vi "Image Display Loop.vi"(11 "Notifier in":refnum<notifier>) -> ()   [LabVIEW 2015]
uses:
  <vilib>/vision/Image Controls.llb/IMAQ Image.ctl
  <vilib>/vision/NI_Vision_Development_Module.lvlib
panel:
  out "Display":T1(plugin-control)
  out "Waveform Graph":T2(graph)
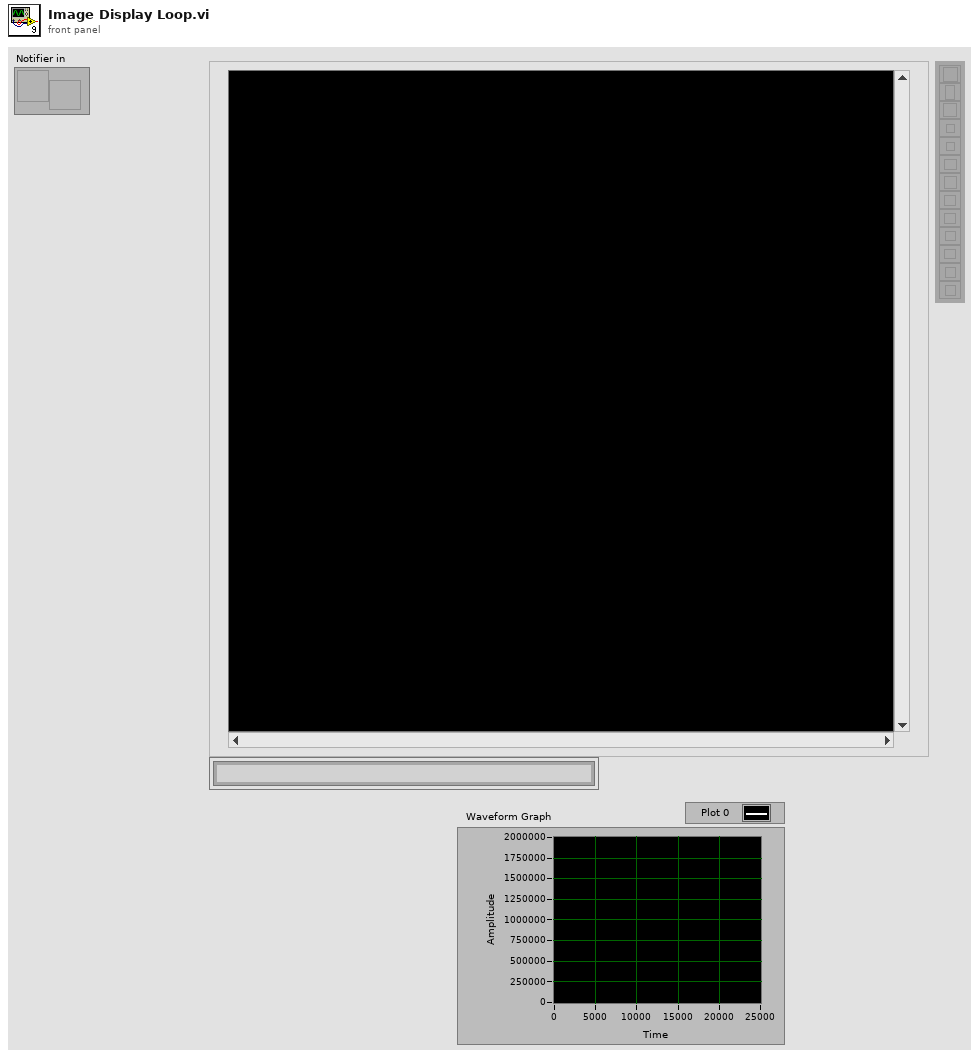
[diagram p1: front panel]
types:
  T1 = typedef "IMAQ Image.ctl" = refnum<image>
  T2 = cluster{"Starting Value":sgl, "Incremental Value":sgl, "Histogram":u32[]}
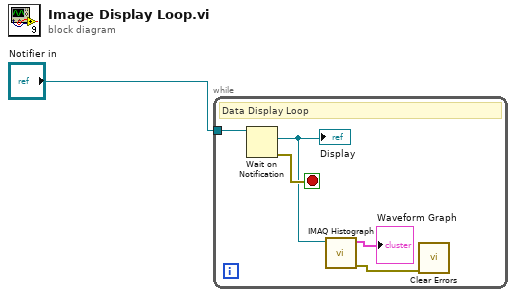
[diagram p0: block diagram]
diagram:
  n1 = while "Data Display Loop" {
    tunnel: "Notifier in" -> [w6]
    stop <- w5 stop-if-true
    # "Data Display Loop"
    n2 = Wait on Notification(notifier=w6) -> (notification=w4:T1, error out=w5:errorcluster)  [unwired: 3 in, 2 out]
    "Display" <- w4
    n3 = call "IMAQ Histograph"("Image"=w4) -> ("error out"=w2:errorcluster, "Histogram Graph"=→"Waveform Graph":T2)  [unwired: 7 in, 2 out]
    n4 = call <vilib>:"Clear Errors.vi"("error in (no error)"=w2) -> ()  [unwired: 5 in, 2 out]
  }
